vi "Calculate Target Data.vi"(7 "X resolution":i32, 8 "Rect Left":dbl, 9 "Rect Right":dbl, 10 "Real size to pixle ratio (in/px)":dbl, 11 "Distance to Target (in)":dbl) -> (2 "X Location (in)":dbl, 3 "Angle":dbl)   [LabVIEW 2012]
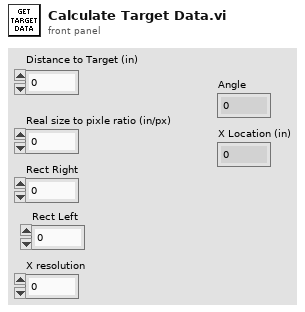
[diagram p1: front panel]
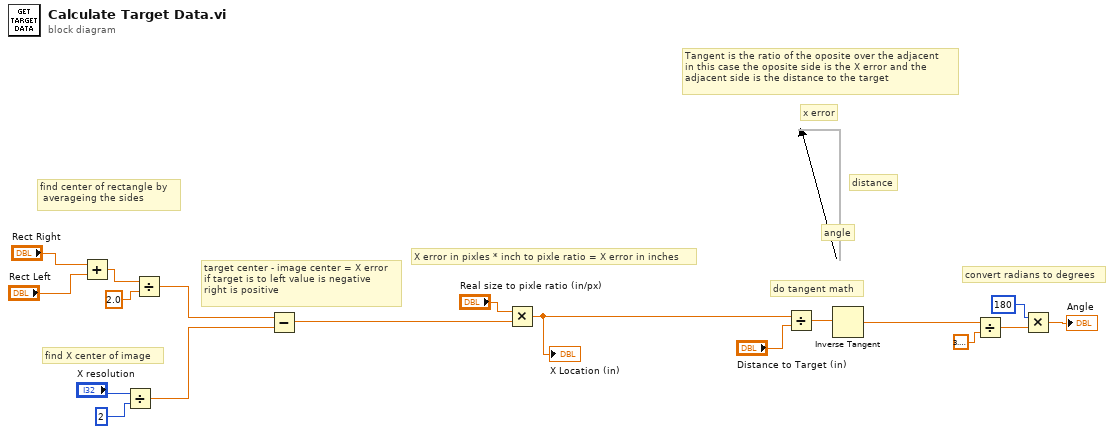
[diagram p0: block diagram]
diagram:
  # "convert radians to degrees"
  # "do tangent math"
  # "angle"
  # "distance"
  # "x error"
  # "Tangent is the ratio of the oposite over the adjacent\nin this case the oposite side is the X error and the\nadjacent side is the distance to the target"
  # "X error in pixles * inch to pixle ratio = X error in inches"
  # "target center - image center = X error\nif target is to left value is negative\nright is positive"
  # "find X center of image"
  # "find center of rectangle by\n averageing the sides"
  n1 = Add(x="Rect Right", y="Rect Left") -> (x+y=w13:dbl)
  n2 = Divide(x="X resolution", y=2) -> (x/y=w9:dbl)
  n3 = Divide(x=w13, y=2.0) -> (x/y=w10:dbl)
  n4 = Subtract(x=w10, y=w9) -> (x-y=w8:dbl)
  n5 = Multiply(x="Real size to pixle ratio (in/px)", y=w8) -> (x*y=w6:dbl)
  "X Location (in)" <- w6
  n6 = Divide(x=w6, y="Distance to Target (in)") -> (x/y=w17:dbl)
  n7 = Inverse Tangent(1:w17) -> (0:w2:dbl)
  n8 = Divide(x=w2, y=3.141592653589793) -> (x/y=w3:dbl)
  n9 = Multiply(x=180, y=w3) -> (x*y=→"Angle":dbl)
